vi "Peak-Valley-Noise.vi"(7 "Pulse":bool, 8 "error in (no error)":errorcluster, 9 "Heart Rate Timer":i32, 10 "Slope":dbl, 11 "Last Slope":dbl) -> (0 "error out":errorcluster, 3 "State":string)   [LabVIEW 2017]
doc: "Peak-Valley-Noise.vi has the following inputs:\ni. Slope - this is the rate at which the pressure is changing between the two most recent points\nii. Last Slope - this is the rate at which the pressure is changing between the previous two points\niii. Heart Rate Timer- this corresponds to the number of data-points that have been analyzed since the previous valley. If the number of samples is less than 300, it should return 'Noise'\niv. Pulse - set to True after a Valley and until a Peak\nv. error in (no error) - if an error is passed into this VI, it should return the same error and zeros for both indicators.\n\nPeak-Valley-Noise.vi has the following outputs:\ni. State - the options are Peak, Valley or Noise\nii. error out - if invalid inputs are received by this VI, it will output an error. It will also pass any errors that are input to it."
panel:
  # "INPUTS"
  # "OUTPUTS"
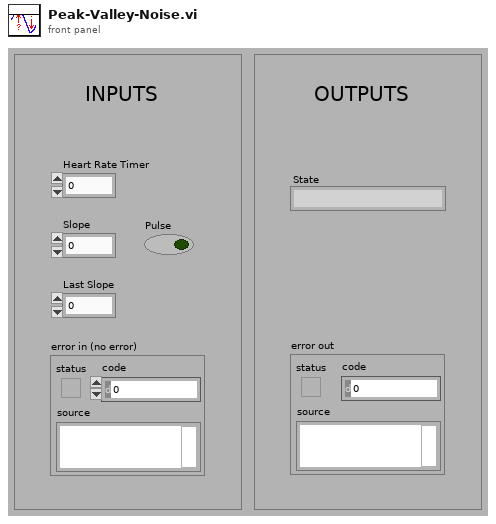
[diagram p1: front panel]
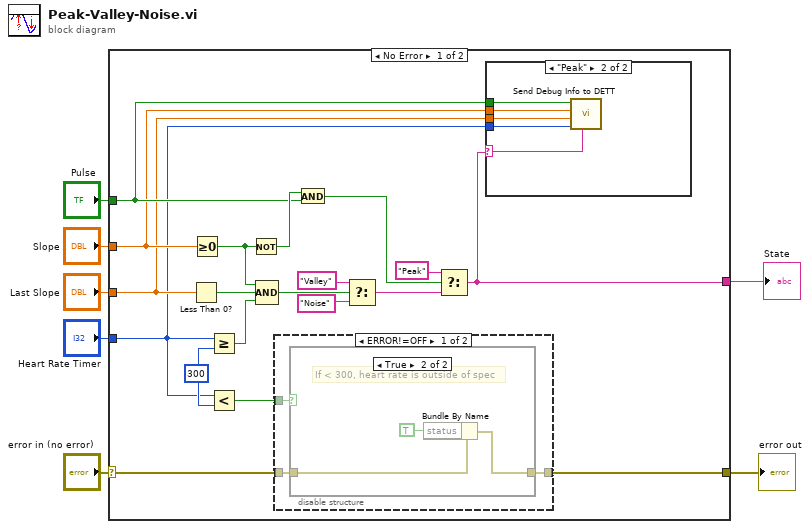
[diagram p0: block diagram]
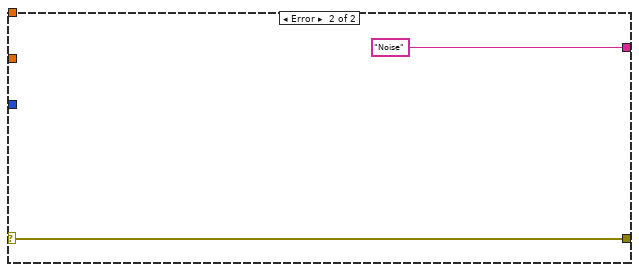
[diagram p5: hidden frame]
diagram:
  n1 = case shown="No Error" "error in (no error)" {
    selector: "error in (no error)" -> [w14 w41]
    tunnel: "Slope" -> [w11 _]
    tunnel: "Last Slope" -> [w10 _]
    tunnel: "Pulse" -> [w12 _]
    tunnel: "Heart Rate Timer" -> [w9 _]
    tunnel: [w8 "Noise" ("f")] -> w3
    tunnel: [w13 w41] -> w1
    frame No Error {
      w16 = 300 ("y")
      n2 = Less Than 0?(x=w10) -> (x < 0?=w18:bool)
      n3 = Greater Or Equal To 0?(x=w11) -> (x >= 0?=w22:bool)
      n4 = Greater Or Equal?(x=w9, y=w16) -> (x >= y?=w17:bool)
      n5 = Less?(x=w9, y=w16) -> (x < y?=w15:bool)
      n6 = Not(x=w22) -> (.not. x?=w23:bool)
      n7 = Compound Arithmetic op=AND(w22, w18, w17) -> (w19:bool)
      n8 = disable-structure shown="ERROR!=OFF" {
        disable-tunnel: w15 -> [w34 _]
        disable-tunnel: w14 -> [w33 w39]
        disable-tunnel: [w32 w39] -> w13
        frame condition #0 {
          n9 = case shown="True" w34 {
            tunnel: w33 -> [w35 w37]
            tunnel: [w35 w36] -> w32
            frame False {
            }
            frame True {
              # "If < 300, heart rate is outside of spec"
              n10 = Bundle By Name(cluster=w37, "status"=TRUE) -> (w36:errorcluster)
            }
          }
        }
        frame condition #1 (active) {
        }
      }
      n11 = And(x=w23, y=w12) -> (x .and. y?=w24:bool)
      n12 = Select(t="Valley", s=w19, f="Noise") -> (s? t:f=w26:string)
      n13 = Select(t="Peak", s=w24, f=w26) -> (s? t:f=w8:string)
      n14 = case shown="\"Peak\"" w8 {
        selector: w8 -> [_ w27]
        tunnel: w12 -> [_ w31]
        tunnel: w11 -> [_ w30]
        tunnel: w10 -> [_ w29]
        tunnel: w9 -> [_ w28]
        frame Default {
        }
        frame "Peak" {
          n15 = call "Send Debug Info to DETT.vi"("f"=w27, "Heart Rate Timer"=w28, "Last Slope"=w29, "Slope"=w30, "Pulse"=w31) -> ()  [unwired: 7 in]
        }
      }
    }
    frame Error {
    }
  }
  "State" <- w3
  "error out" <- w1
